vi "autofpga8.vi"() -> ()   [LabVIEW 2012]
uses:
  <vilib>/eio/EIONode/EIONode.xnode
  <vilib>/eio/EIOMethodNode/EIOMethodNode.xnode
  <vilib>/LabVIEW Targets/FPGA/RIO/nicrio_985x_controls.llb/CAN_IO_Frame Type.ctl
  <vilib>/LabVIEW Targets/FPGA/RIO/nicrio_985x_controls.llb/CAN_IO_Frame Cluster.ctl
  <vilib>/rvi/eio/common/nirviEmuTemplateMethod_errors.vi
  <vilib>/eio/EIOPropertyNode/EIOPropertyNode.xnode
  <vilib>/rvi/eio/common/nirviEmuTemplatePropertyGet_errors.vi
  <vilib>/rvi/eio/common/nirviEmuTemplatePropertyGet_noerrors.vi
  <vilib>/rvi/eio/common/nirviEmuTemplatePropertySet_errors.vi
  <vilib>/rvi/eio/common/nirviEmuTemplatePropertySet_noerrors.vi
  <vilib>/rvi/DataTransferAndStorage/Container/XNode/niFpgaContainer.xnode
  <vilib>/rvi/interface/RandomDataEmulation/nirviRandomDataFpgaReadWriteTemplate.vi
panel:
  out "Data":u8
  out "Is gps1 Connected":bool
  out "Connection error GPS 1":bool=TRUE
  out "GPS 1 clock":bool=TRUE
  out "DATA IMU 1":T1
  out "IMU Connection error":bool=TRUE
  out "Idle rpm":u8
  out "ODOMETERT_RL":u8
  out "WHEEL_FR":u8
  out "WHEEL_FRFL":u8
  out "WHEEL_FL":u8
  in  "16k":bool
  out "amp":fxp<+/-,16,5> format="%.13g"
  out "WHELL_RR":u8
  out "WHEEL_RRRL":u8
  out "WHEEL_RL":u8
  out "counter":bool=TRUE
  out "lock on":bool
  out "rpm":u16
  out "BREAK_ACT_TCU":u8
  out "VS_TCU 2":u8
  out "VS_TCU":u8
  out "VB":u8
  out "TPS":u8
  out "Vehicle speed":u8
  out "G_sel_disp":u8
  out "SAS_angle":i32
  out "SAS_angle_MDPS":i32
  out "OPT1_Read":bool
  in  "OPT1_Write":bool
  in  "OPT1_write enable":bool
  out "encoder":u16
  out "T Lim":bool
  in  "Buzz":bool
  out "CAN read":T2={"timestamp high"=0, "timestamp low"=0, "identifier"=0, "type"=enum."Data Frame", "info A"=0, "info B"=0, "data length"=0, "data"=[0, 0, 0, 0, 0, 0, 0, 0]} {"identifier" format="%x"; "timestamp high" format="%08x"; "timestamp low" format="%08x"; "data" format="%.0x"}
  in  "CAN Write":T2={"timestamp high"=0, "timestamp low"=0, "identifier"=1540, "type"=enum."Data Frame", "info A"=0, "info B"=0, "data length"=8, "data"=[0, 0, 0, 0, 0, 0, 0, 0]} {"identifier" format="%x"; "timestamp high" format="%08x"; "timestamp low" format="%08x"; "data" format="%.0x"}
  in  "read can":bool
  in  "B Pwm":u16
  in  "T Pwm":u16
  in  "Shift PWM":bool
  in  "B Dir":bool
  in  "B RDir":bool
  in  "Shift Dir":bool
  in  "T Dir":bool
  in  "T RDir":bool
  in  "Solenoid":bool
  out "Run":bool
  out "Auto":bool
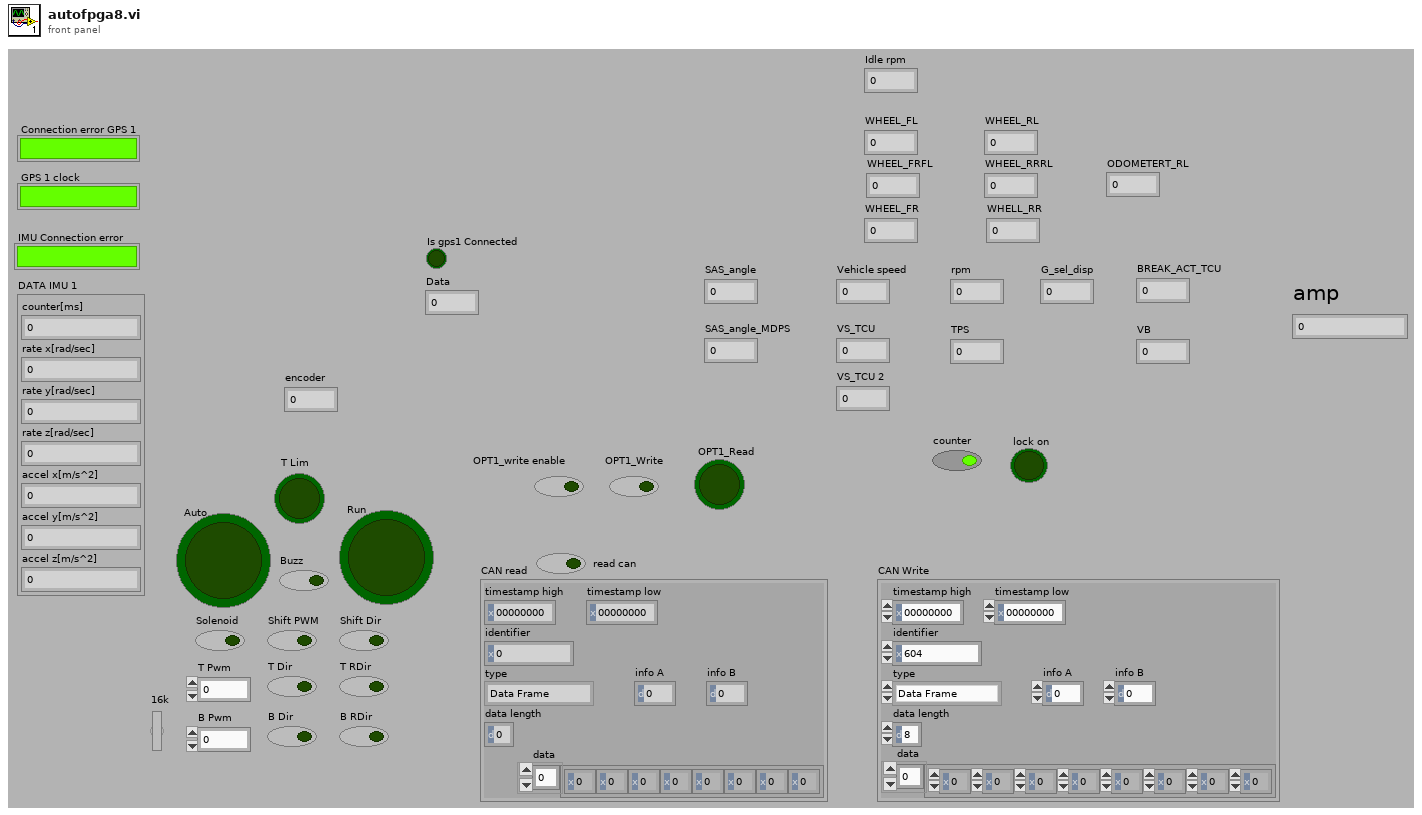
[diagram p1: front panel]
types:
  T1 = cluster{"counter[ms]":u16, "rate x[rad/sec]":i16, "rate y[rad/sec]":i16, "rate z[rad/sec]":i16, "accel x[m/s^2]":i16, "accel y[m/s^2]":i16, "accel z[m/s^2]":i16}
  T2 = typedef "CAN_IO_Frame Cluster.ctl" = cluster{"timestamp high":u32, "timestamp low":u32, "identifier":u32, "type":T3, "info A":u8, "info B":u8, "data length":u8, "data":u8[]}
  T3 = typedef "CAN_IO_Frame Type.ctl" = enum8{"Data Frame", "Remote Frame", "(reserved)", "(reserved) ", "(reserved)  ", "(reserved)   ", "Bus Error", "Transceiver Fault"}
  T4 = cluster{"data[0]":u8, "data[1]":u8, "data[2]":u8, "data[3]":u8, "data[4]":u8, "data[5]":u8, "data[6]":u8, "data[7]":u8}
  T5 = cluster{"[0]":void, "[1]":void, "[2]":void, "[3]":void, "[4]":void, "[5]":void, "[6]":void, "[7]":void, "[8]":void, "[9]":void, "[10]":void, "[11]":void, "[12]":void, "[13]":void}
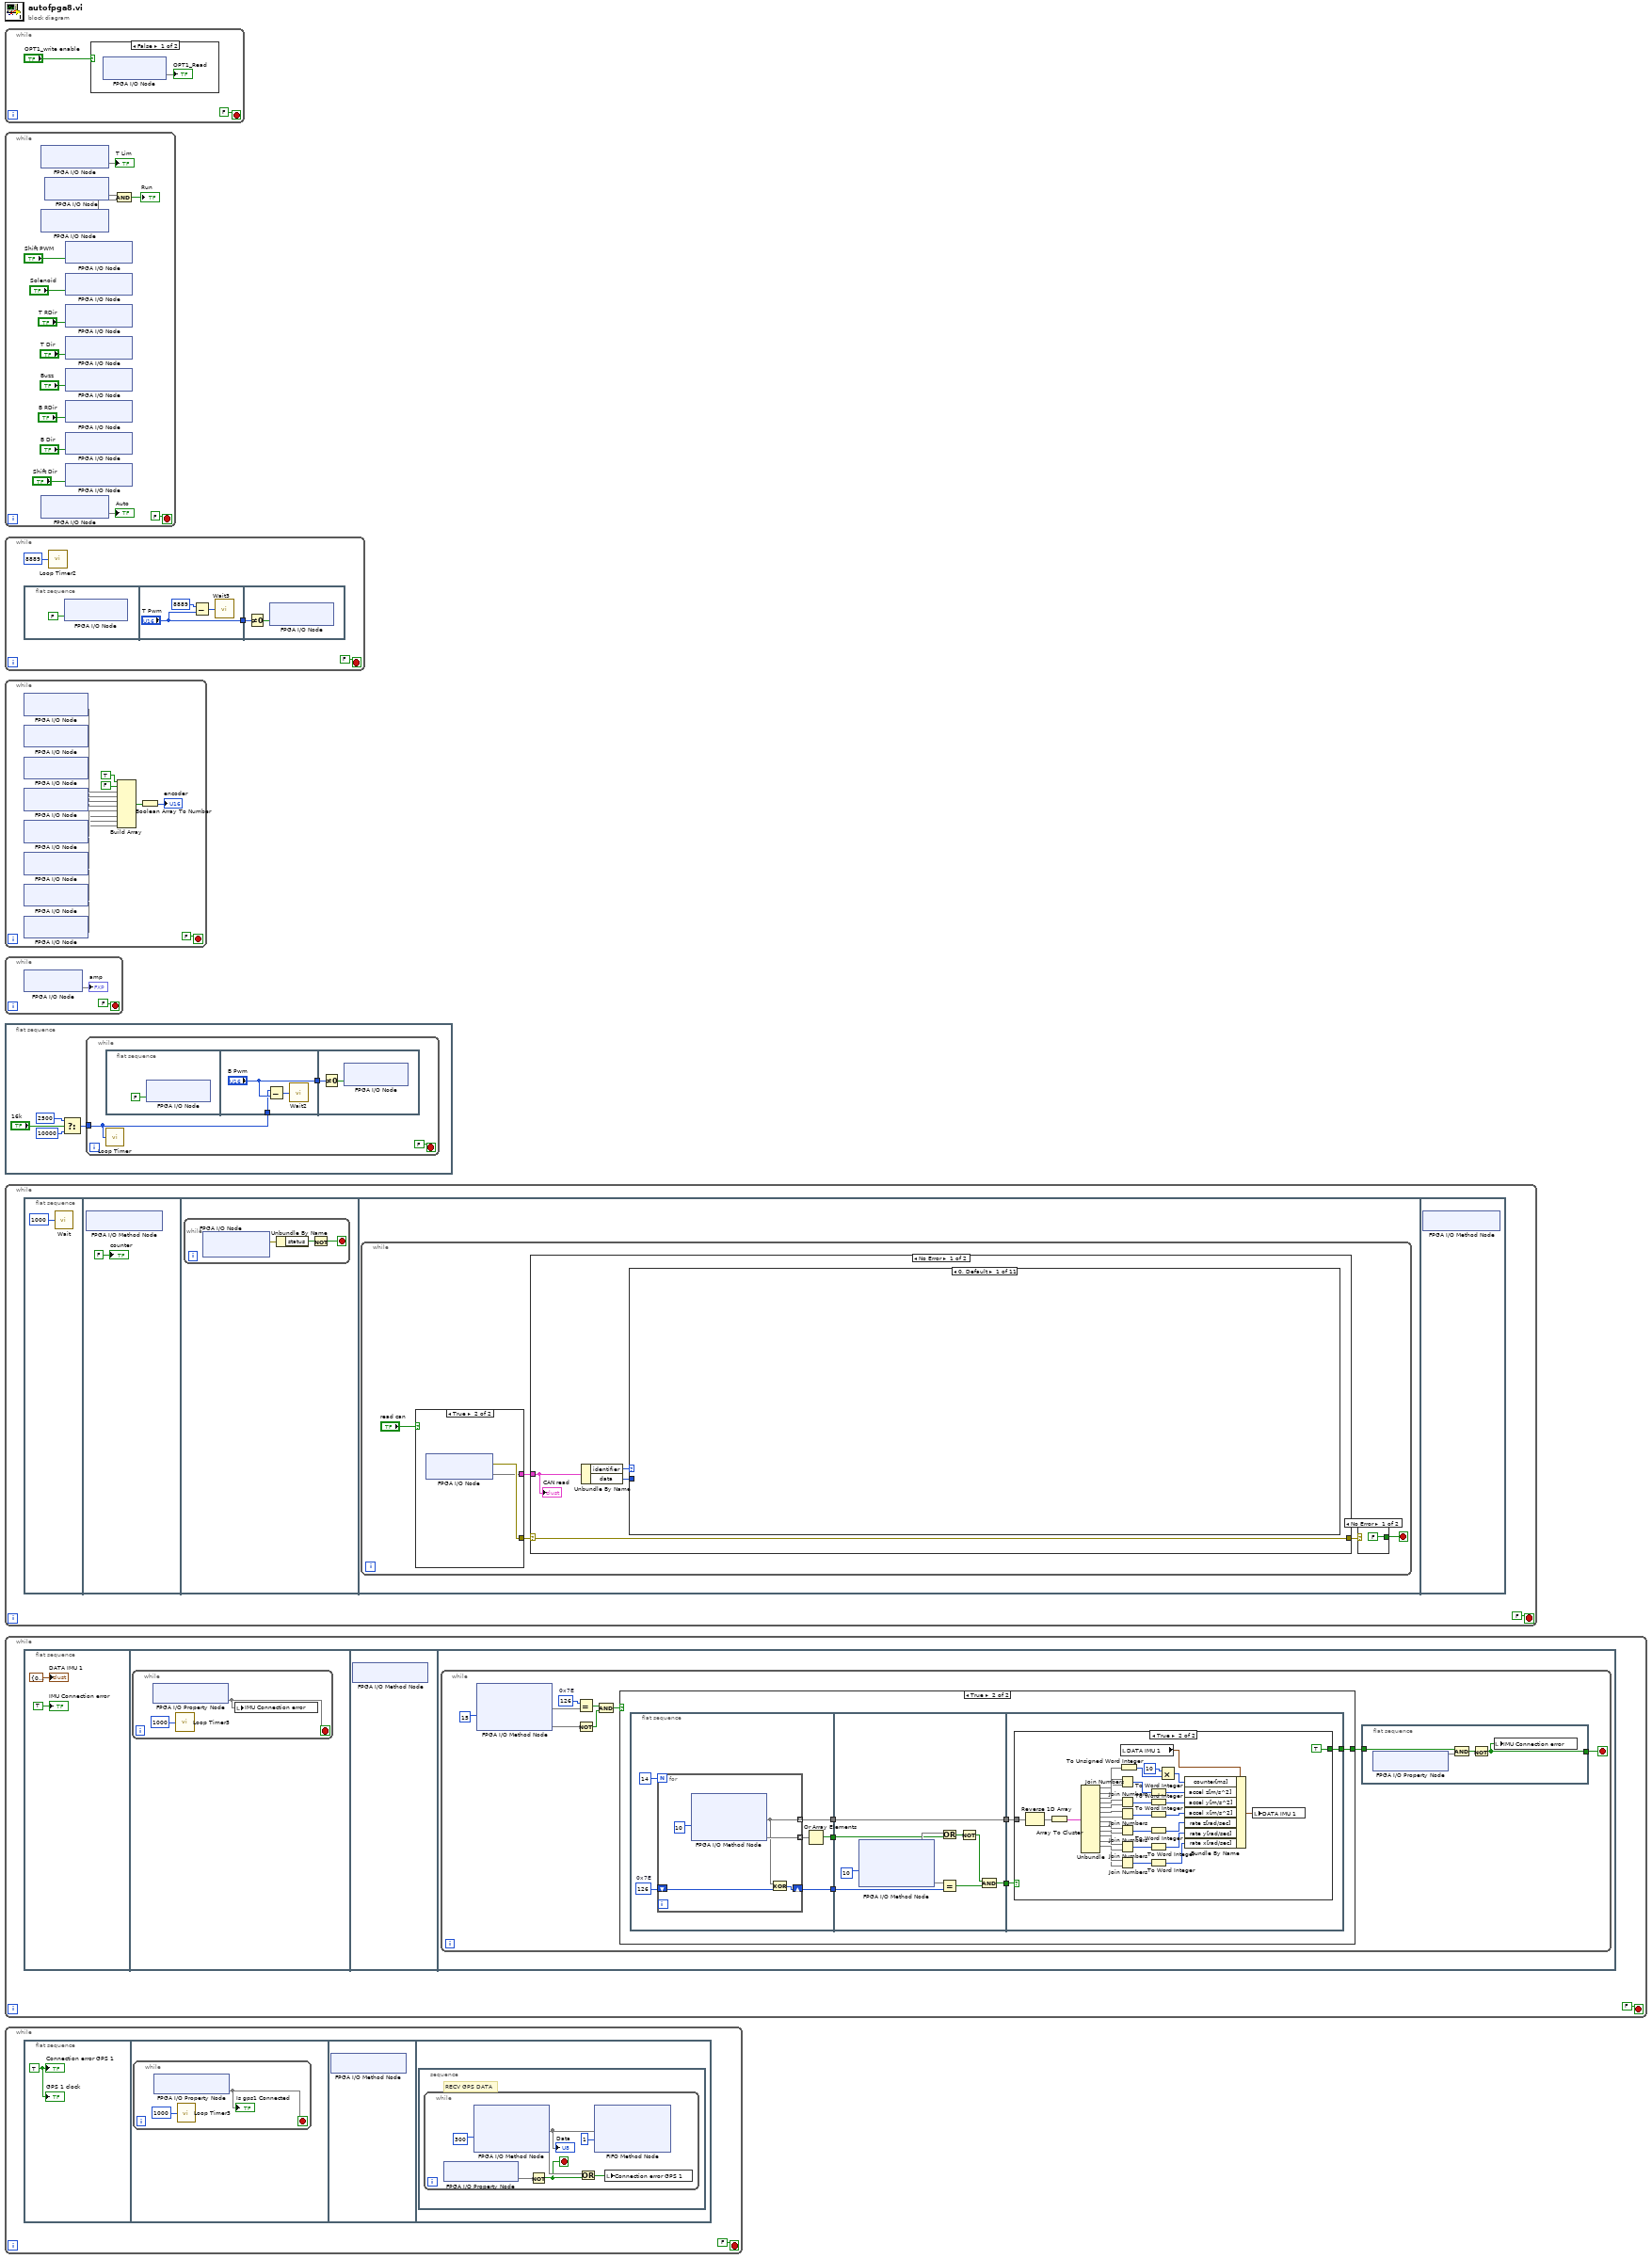
[diagram p0: block diagram]
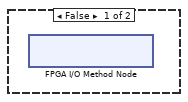
[diagram p3: hidden frame]
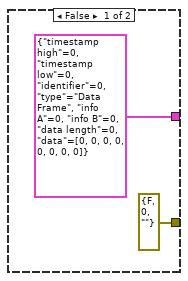
[diagram p4: hidden frame]
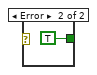
[diagram p5: hidden frame]
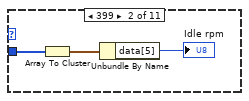
[diagram p6: hidden frame]
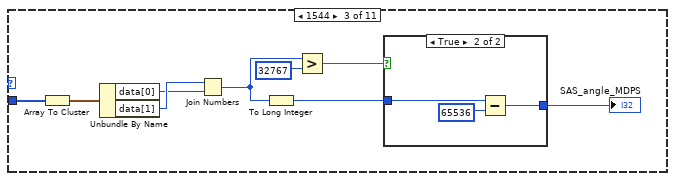
[diagram p7: hidden frame]
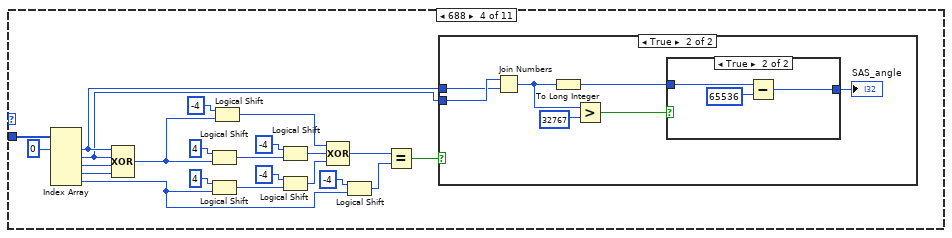
[diagram p9: hidden frame]
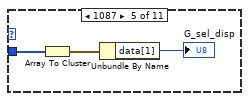
[diagram p12: hidden frame]
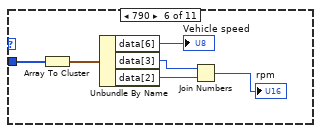
[diagram p13: hidden frame]
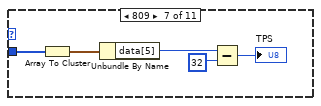
[diagram p14: hidden frame]
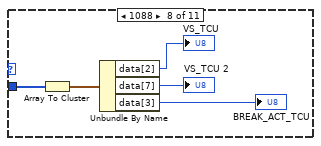
[diagram p15: hidden frame]
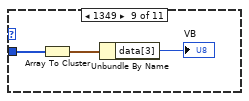
[diagram p16: hidden frame]
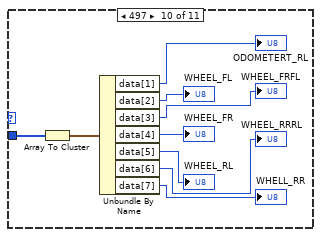
[diagram p17: hidden frame]
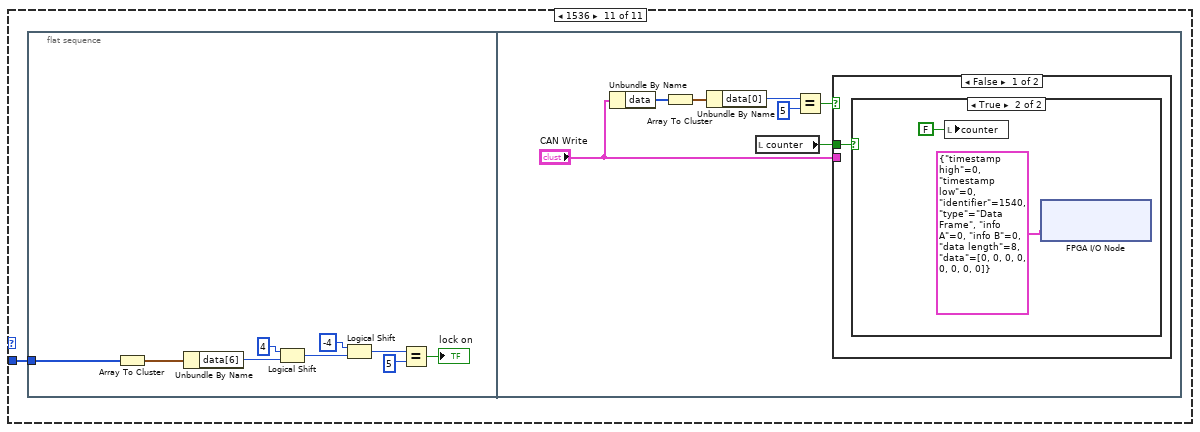
[diagram p18: hidden frame]
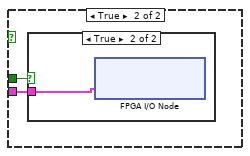
[diagram p20: hidden frame]
diagram:
  n1 = while {
    stop <- FALSE stop-if-true
    n2 = case shown="False" "OPT1_write enable" {
      frame False {
        n3 = xnode "FPGA I/O Node"() -> ("Mod1/DIO0"=→"OPT1_Read")  [unwired: 1 in, 1 out]
      }
      frame True {
        n4 = xnode "FPGA I/O Node"("Mod1/DIO0"="OPT1_Write") -> ()  [unwired: 1 in, 1 out]
      }
    }
  }
  n5 = while {
    stop <- FALSE stop-if-true
    n6 = xnode "FPGA I/O Node"() -> ("Mod1/DIO15"=→"T Lim")  [unwired: 1 in, 1 out]
    n7 = xnode "FPGA I/O Node"() -> ("Mod1/DIO12"=w7)  [unwired: 1 in, 1 out]
    n8 = xnode "FPGA I/O Node"() -> ("Mod1/DIO11"=→"Auto")  [unwired: 1 in, 1 out]
    n9 = xnode "FPGA I/O Node"() -> ("Mod1/DIO0"=w8)  [unwired: 1 in, 1 out]
    n10 = xnode "FPGA I/O Node"("Mod1/DIO19"="Shift PWM") -> ()  [unwired: 1 in, 1 out]
    n11 = xnode "FPGA I/O Node"("Mod1/DIO13"="Solenoid") -> ()  [unwired: 1 in, 1 out]
    n12 = xnode "FPGA I/O Node"("Mod1/DIO17"="T RDir") -> ()  [unwired: 1 in, 1 out]
    n13 = xnode "FPGA I/O Node"("Mod1/DIO18"="T Dir") -> ()  [unwired: 1 in, 1 out]
    n14 = xnode "FPGA I/O Node"("Mod1/DIO24"="Buzz") -> ()  [unwired: 1 in, 1 out]
    n15 = xnode "FPGA I/O Node"("Mod1/DIO22"="B RDir") -> ()  [unwired: 1 in, 1 out]
    n16 = xnode "FPGA I/O Node"("Mod1/DIO23"="B Dir") -> ()  [unwired: 1 in, 1 out]
    n17 = xnode "FPGA I/O Node"("Mod1/DIO20"="Shift Dir") -> ()  [unwired: 1 in, 1 out]
    n18 = And(x=w8, y=w7) -> (x .and. y?=→"Run":bool)
  }
  n19 = while {
    stop <- FALSE stop-if-true
    n20 = flat-sequence {
      tunnel: ["T Pwm"] -> w19
      tunnel: w19 -> [w27]
      frame #0 {
        n21 = xnode "FPGA I/O Node"("Mod4/DIO1"=FALSE ("Mod1/DIO16")) -> ()  [unwired: 1 in, 1 out]
      }
      frame #1 {
        n22 = Subtract(x=u16 8889, y="T Pwm") -> (x-y=w24:u16)
        n23 = call "Wait3"("Count(Ticks)"=w24) -> ()  [unwired: 1 out]
      }
      frame #2 {
        n24 = Not Equal To 0?(x=w27) -> (x != 0?=w26:bool)
        n25 = xnode "FPGA I/O Node"("Mod4/DIO1"=w26) -> ()  [unwired: 1 in, 1 out]
      }
    }
    n26 = call "Loop Timer2"("Count(Ticks)"=u16 8889) -> ()  [unwired: 1 out]
  }
  n27 = while {
    stop <- FALSE stop-if-true
    n28 = xnode "FPGA I/O Node"() -> ("Mod1/DIO2"=w40)  [unwired: 1 in, 1 out]
    n29 = xnode "FPGA I/O Node"() -> ("Mod1/DIO3"=w39)  [unwired: 1 in, 1 out]
    n30 = xnode "FPGA I/O Node"() -> ("Mod1/DIO4"=w38)  [unwired: 1 in, 1 out]
    n31 = xnode "FPGA I/O Node"() -> ("Mod1/DIO5"=w37)  [unwired: 1 in, 1 out]
    n32 = xnode "FPGA I/O Node"() -> ("Mod1/DIO6"=w36)  [unwired: 1 in, 1 out]
    n33 = xnode "FPGA I/O Node"() -> ("Mod1/DIO7"=w35)  [unwired: 1 in, 1 out]
    n34 = xnode "FPGA I/O Node"() -> ("Mod1/DIO8"=w34)  [unwired: 1 in, 1 out]
    n35 = xnode "FPGA I/O Node"() -> ("Mod1/DIO9"=w33)  [unwired: 1 in, 1 out]
    n36 = Build Array(TRUE ("element"), FALSE ("element"), w40, w39, w38, w37, w36, w35, w34, w33) -> (w31:bool[])
    n37 = Boolean Array To Number(Boolean array=w31) -> (number=→"encoder":u32)
  }
  n38 = while {
    stop <- FALSE stop-if-true
    n39 = xnode "FPGA I/O Node"() -> ("Mod3/AI7"=→"amp")  [unwired: 1 in, 1 out]
  }
  n40 = flat-sequence {
    frame #0 {
      n41 = Select(t=u16 2500, s="16k", f=u16 10000) -> (s? t:f=w43:u16)
      n42 = while {
        tunnel: w43 -> [w47]
        stop <- FALSE stop-if-true
        n43 = flat-sequence {
          tunnel: ["B Pwm"] -> w49
          tunnel: w47 -> [w51]
          tunnel: w49 -> [w55]
          frame #0 {
            n44 = xnode "FPGA I/O Node"("Mod4/DIO0"=FALSE ("Mod1/DIO21")) -> ()  [unwired: 1 in, 1 out]
          }
          frame #1 {
            n45 = Subtract(x=w51, y="B Pwm") -> (x-y=w53:u16)
            n46 = call "Wait2"("Count(Ticks)"=w53) -> ()  [unwired: 1 out]
          }
          frame #2 {
            n47 = Not Equal To 0?(x=w55) -> (x != 0?=w54:bool)
            n48 = xnode "FPGA I/O Node"("Mod4/DIO0"=w54) -> ()  [unwired: 1 in, 1 out]
          }
        }
        n49 = call "Loop Timer"("Count(Ticks)"=w47) -> ()  [unwired: 1 out]
      }
    }
  }
  n50 = while {
    stop <- FALSE stop-if-true
    n51 = flat-sequence {
      frame #0 {
        n52 = call "Wait"("Count(mSec)"=u16 1000) -> ()  [unwired: 1 out]
      }
      frame #1 {
        n53 = xnode "FPGA I/O Method Node"() -> ()  [unwired: 2 in, 2 out]
        "counter" <- FALSE
      }
      frame #2 {
        n54 = while {
          stop <- w59 stop-if-true
          n55 = xnode "FPGA I/O Node"() -> ("error out"=w61:errorcluster)  [unwired: 2 in, 2 out]
          n56 = Unbundle By Name(w61) -> ("status"=w60:bool)
          n57 = Not(x=w60) -> (.not. x?=w59:bool)
        }
      }
      frame #3 {
        n58 = while {
          stop <- w62 stop-if-true
          n59 = case shown="True" "read can" {
            tunnel: [errorcluster {"status"=FALSE, "code"=0, "source"=""} ("error out") w70] -> w66
            tunnel: [T2 {"timestamp high"=0, "timestamp low"=0, "identifier"=0, "type"=enum."Data Frame", "info A"=0, "info B"=0, "data length"=0, "data"=[0, 0, 0, 0, 0, 0, 0, 0]} ("Mod3/CAN0") w69] -> w65
            frame False {
            }
            frame True {
              n60 = xnode "FPGA I/O Node"() -> ("error out"=w70:errorcluster, "Mod2/CAN0"=w69)  [unwired: 2 in, 1 out]
            }
          }
          n61 = case shown="No Error" w66 {
            selector: w66 -> [w73 w181]
            tunnel: w65 -> [w76 _]
            tunnel: [w73 w181] -> w64
            frame No Error {
              n62 = Unbundle By Name(w76) -> ("identifier"=w75:u32, "data"=w74:u8[])
              n63 = case shown="0, Default" w75 {
                tunnel: w74 -> [_ w78 w87 w93 w128 w133 w138 w143 w146 w155 w157]
                frame 0, Default {
                }
                frame 399 {
                  n64 = Array To Cluster(array=w78) -> (cluster=w79:T4)
                  n65 = Unbundle By Name(w79) -> ("data[5]"=→"Idle rpm":u8)
                }
                frame 1544 {
                  n66 = Array To Cluster(array=w87) -> (cluster=w88:T4)
                  n67 = Unbundle By Name(w88) -> ("data[0]"=w85:u8, "data[1]"=w86:u8)
                  n68 = Join Numbers(hi=w86, lo=w85) -> ((hi.lo)=w82:u16)
                  n69 = To Long Integer(number=w82) -> (32bit integer=w81:i32)
                  n70 = Greater?(x=w82, y=u16 32767) -> (0:w83:bool)
                  n71 = case shown="True" w83 {
                    tunnel: w81 -> [w89 w90]
                    tunnel: [w89 w91] -> w80
                    frame False {
                    }
                    frame True {
                      n72 = Subtract(x=w90, y=65536) -> (x-y=w91:i32)
                    }
                  }
                  "SAS_angle_MDPS" <- w80
                }
                frame 688 {
                  n73 = Index Array(array=w93, index #1=0 ("index")) -> (element #1=w98:u8, element #2=w97:u8, element #3=w96:u8, element #4=w95:u8, element #5=w94:u8)  [unwired: 4 in]
                  n74 = Compound Arithmetic op=XOR(w98, w97, w96, w95) -> (w114:u8)
                  n75 = Logical Shift(y=i8 4, x=w114) -> (x << y=w113:u8)
                  n76 = Logical Shift(y=i8 4, x=w94) -> (x << y=w106:u8)
                  n77 = Logical Shift(y=i8 -4, x=w114) -> (x << y=w107:u8)
                  n78 = Logical Shift(y=i8 -4, x=w113) -> (x << y=w108:u8)
                  n79 = Logical Shift(y=i8 -4, x=w106) -> (x << y=w101:u8)
                  n80 = Compound Arithmetic op=XOR(w107, w108, w101) -> (w109:u8)
                  n81 = Logical Shift(y=i8 -4, x=w94) -> (x << y=w102:u8)
                  n82 = Equal?(x=w109, y=w102) -> (x = y?=w100:bool)
                  n83 = case shown="True" w100 {
                    tunnel: w97 -> [_ w121]
                    tunnel: w98 -> [_ w120]
                    frame False {
                    }
                    frame True {
                      n84 = Join Numbers(hi=w121, lo=w120) -> ((hi.lo)=w117:u16)
                      n85 = To Long Integer(number=w117) -> (32bit integer=w116:i32)
                      n86 = Greater?(x=w117, y=u16 32767) -> (0:w118:bool)
                      n87 = case shown="True" w118 {
                        tunnel: w116 -> [w122 w124]
                        tunnel: [w122 w123] -> w115
                        frame False {
                        }
                        frame True {
                          n88 = Subtract(x=w124, y=65536) -> (x-y=w123:i32)
                        }
                      }
                      "SAS_angle" <- w115
                    }
                  }
                }
                frame 1087 {
                  n89 = Array To Cluster(array=w128) -> (cluster=w127:T4)
                  n90 = Unbundle By Name(w127) -> ("data[1]"=→"G_sel_disp":u8)
                }
                frame 790 {
                  n91 = Array To Cluster(array=w133) -> (cluster=w134:T4)
                  n92 = Unbundle By Name(w134) -> ("data[6]"=→"Vehicle speed":u8, "data[3]"=w131:u8, "data[2]"=w130:u8)
                  n93 = Join Numbers(hi=w131, lo=w130) -> ((hi.lo)=→"rpm":u16)
                }
                frame 809 {
                  n94 = Array To Cluster(array=w138) -> (cluster=w139:T4)
                  n95 = Unbundle By Name(w139) -> ("data[5]"=w137:u8)
                  n96 = Subtract(x=w137, y=u8 32) -> (x-y=→"TPS":u8)
                }
                frame 1088 {
                  n97 = Array To Cluster(array=w143) -> (cluster=w144:T4)
                  n98 = Unbundle By Name(w144) -> ("data[2]"=→"VS_TCU":u8, "data[7]"=→"VS_TCU 2":u8, "data[3]"=→"BREAK_ACT_TCU":u8)
                }
                frame 1349 {
                  n99 = Array To Cluster(array=w146) -> (cluster=w147:T4)
                  n100 = Unbundle By Name(w147) -> ("data[3]"=→"VB":u8)
                }
                frame 497 {
                  n101 = Array To Cluster(array=w155) -> (cluster=w156:T4)
                  n102 = Unbundle By Name(w156) -> ("data[1]"=→"ODOMETERT_RL":u8, "data[2]"=→"WHEEL_FL":u8, "data[3]"=→"WHEEL_FRFL":u8, "data[4]"=→"WHEEL_FR":u8, "data[5]"=→"WHEEL_RL":u8, "data[6]"=→"WHEEL_RRRL":u8, "data[7]"=→"WHELL_RR":u8)
                }
                frame 1536 {
                  n103 = flat-sequence {
                    tunnel: w157 -> [w166]
                    frame #0 {
                      n104 = Array To Cluster(array=w166) -> (cluster=w165:T4)
                      n105 = Unbundle By Name(w165) -> ("data[6]"=w164:u8)
                      n106 = Logical Shift(y=i8 4, x=w164) -> (x << y=w163:u8)
                      n107 = Logical Shift(y=i8 -4, x=w163) -> (x << y=w160:u8)
                      n108 = Equal?(x=w160, y=u8 5) -> (x = y?=→"lock on":bool)
                    }
                    frame #1 {
                      n109 = Unbundle By Name("CAN Write") -> ("data"=w171:u8[])
                      n110 = Array To Cluster(array=w171) -> (cluster=w170:T4)
                      n111 = Unbundle By Name(w170) -> ("data[0]"=w169:u8)
                      n112 = local read "counter"() -> (w167:bool)
                      n113 = Equal?(x=w169, y=u8 5) -> (x = y?=w173:bool)
                      n114 = case shown="False" w173 {
                        tunnel: "CAN Write" -> [_ w178]
                        tunnel: w167 -> [w174 w177]
                        frame False {
                          n115 = case shown="True" w174 {
                            frame False {
                            }
                            frame True {
                              n116 = local write "counter"(FALSE ("counter")) -> ()
                              n117 = xnode "FPGA I/O Node"("Mod2/CAN0"=T2 {"timestamp high"=0, "timestamp low"=0, "identifier"=1540, "type"=enum."Data Frame", "info A"=0, "info B"=0, "data length"=8, "data"=[0, 0, 0, 0, 0, 0, 0, 0]} ("CAN Write")) -> ()  [unwired: 2 in, 2 out]
                            }
                          }
                        }
                        frame True {
                          n118 = case shown="True" w177 {
                            tunnel: w178 -> [_ w180]
                            frame False {
                              n119 = local write "counter"(TRUE ("counter")) -> ()
                            }
                            frame True {
                              n120 = xnode "FPGA I/O Node"("Mod2/CAN0"=w180) -> ()  [unwired: 2 in, 2 out]
                            }
                          }
                        }
                      }
                    }
                  }
                }
              }
              "CAN read" <- w76
            }
            frame Error {
            }
          }
          n121 = case shown="No Error" w64 {
            tunnel: [FALSE ("can_ini") TRUE ("can_ini")] -> w62
            frame No Error {
            }
            frame Error {
            }
          }
        }
      }
      frame #4 {
        n122 = xnode "FPGA I/O Method Node"() -> ()  [unwired: 2 in, 2 out]
      }
    }
  }
  n123 = while {
    stop <- FALSE stop-if-true
    n124 = flat-sequence {
      frame #0 {
        "DATA IMU 1" <- T1 {"counter[ms]"=0, "rate x[rad/sec]"=0, "rate y[rad/sec]"=0, "rate z[rad/sec]"=0, "accel x[m/s^2]"=0, "accel y[m/s^2]"=0, "accel z[m/s^2]"=0} ("DATA IMU 1")
        "IMU Connection error" <- TRUE ("IMU Connection error")
      }
      frame #1 {
        n125 = while {
          stop <- w185 stop-if-true
          n126 = xnode "FPGA I/O Property Node"() -> ("Is Connected"=w185)  [unwired: 1 in, 1 out]
          n127 = call "Loop Timer5"("Count(mSec)"=u32 1000) -> ()  [unwired: 1 out]
          n128 = local write "IMU Connection error"(w185) -> ()
        }
      }
      frame #2 {
        n129 = xnode "FPGA I/O Method Node"() -> ()  [unwired: 1 in, 1 out]
      }
      frame #3 {
        n130 = while {
          stop <- w187 stop-if-true
          w189 = u8 126  # 0x7E
          n131 = xnode "FPGA I/O Method Node"("Timeout (ms)"=15) -> ("Data"=w190, "Timed Out"=w194)  [unwired: 1 in, 1 out]
          n132 = Equal?(x=w189, y=w190) -> (x = y?=w193:bool)
          n133 = Not(x=w194) -> (.not. x?=w192:bool)
          n134 = And(x=w193, y=w192) -> (x .and. y?=w191:bool)
          n135 = case shown="True" w191 {
            tunnel: [_ w201] -> w188
            frame False {
            }
            frame True {
              n136 = flat-sequence {
                tunnel: [w209] -> w205
                tunnel: [w208] -> w203
                tunnel: [w206] -> w200
                tunnel: w205 -> [w226]
                tunnel: [w226] -> w204
                tunnel: w203 -> [w219]
                tunnel: [w221] -> w202
                tunnel: w200 -> [w223]
                tunnel: w204 -> [w229]
                tunnel: w202 -> [w228]
                tunnel: [w227] -> w201
                frame #0 {
                  w210 = u8 126  # 0x7E
                  n137 = for {
                    N: 14 -> [_]
                    tunnel: [w213] -> w209 mode=indexing
                    shift-right: [w215] -> w208
                    shift-left: w210 -> [w212]
                    tunnel: [w214] -> w207 mode=indexing
                    n138 = xnode "FPGA I/O Method Node"("Timeout (ms)"=10) -> ("Data"=w213, "Timed Out"=w214)  [unwired: 1 in, 1 out]
                    n139 = Exclusive Or(1:w212, 2:w213) -> (0:w215:u8)
                  }
                  n140 = Or Array Elements(Boolean array=w207) -> (logical OR=w206:bool)
                }
                frame #1 {
                  n141 = xnode "FPGA I/O Method Node"("Timeout (ms)"=10) -> ("Data"=w220, "Timed Out"=w224)  [unwired: 1 in, 1 out]
                  n142 = Or(x=w224, y=w223) -> (x .or. y?=w222:bool)
                  n143 = Equal?(x=w220, y=w219) -> (x = y?=w218:bool)
                  n144 = Not(x=w222) -> (.not. x?=w217:bool)
                  n145 = And(x=w217, y=w218) -> (x .and. y?=w221:bool)
                }
                frame #2 {
                  n146 = case shown="True" w228 {
                    tunnel: w229 -> [_ w263]
                    tunnel: [_ TRUE ("IMU Connection error")] -> w227
                    frame False {
                      n147 = xnode "FPGA I/O Method Node"() -> ()  [unwired: 1 in, 1 out]
                    }
                    frame True {
                      n148 = Reverse 1D Array(array=w263) -> (reversed array=w262:void[])
                      n149 = Array To Cluster(array=w262) -> (cluster=w261:T5)
                      n150 = Unbundle(w261) -> ("[0]"=w240, "[1]"=w260, "[2]"=w259, "[3]"=w258, "[4]"=w257, "[5]"=w256, "[6]"=w255, "[7]"=w254, "[8]"=w253, "[9]"=w252, "[10]"=w251, "[11]"=w250, "[12]"=w249)  [unwired: 1 out]
                      n151 = Join Numbers(hi=w260, lo=w259) -> ((hi.lo)=w248:u32)
                      n152 = Join Numbers(hi=w258, lo=w257) -> ((hi.lo)=w247:u32)
                      n153 = Join Numbers(hi=w256, lo=w255) -> ((hi.lo)=w246:u32)
                      n154 = Join Numbers(hi=w254, lo=w253) -> ((hi.lo)=w245:u32)
                      n155 = Join Numbers(hi=w252, lo=w251) -> ((hi.lo)=w244:u32)
                      n156 = Join Numbers(hi=w250, lo=w249) -> ((hi.lo)=w243:u32)
                      n157 = To Unsigned Word Integer(number=w240) -> (unsigned 16bit integer=w239:u16)
                      n158 = local read "DATA IMU 1"() -> (w241:T1)
                      n159 = To Word Integer(number=w248) -> (16bit integer=w236:i16)
                      n160 = To Word Integer(number=w247) -> (16bit integer=w235:i16)
                      n161 = To Word Integer(number=w246) -> (16bit integer=w234:i16)
                      n162 = To Word Integer(number=w245) -> (16bit integer=w233:i16)
                      n163 = To Word Integer(number=w244) -> (16bit integer=w232:i16)
                      n164 = To Word Integer(number=w243) -> (16bit integer=w231:i16)
                      n165 = Multiply(x=u16 10, y=w239) -> (x*y=w237:u16)
                      n166 = Bundle By Name(cluster=w241, "counter[ms]"=w237, "accel z[m/s^2]"=w236, "accel y[m/s^2]"=w235, "accel x[m/s^2]"=w234, "rate z[rad/sec]"=w233, "rate y[rad/sec]"=w232, "rate x[rad/sec]"=w231) -> (w242:T1)
                      n167 = local write "DATA IMU 1"(w242) -> ()
                    }
                  }
                }
              }
            }
          }
          n168 = flat-sequence {
            tunnel: w188 -> [w198]
            tunnel: [w196] -> w187
            frame #0 {
              n169 = xnode "FPGA I/O Property Node"() -> ("Is Connected"=w199)  [unwired: 1 in, 1 out]
              n170 = And(x=w198, y=w199) -> (x .and. y?=w197:bool)
              n171 = Not(x=w197) -> (.not. x?=w196:bool)
              n172 = local write "IMU Connection error"(w196) -> ()
            }
          }
        }
      }
    }
  }
  n173 = while {
    stop <- FALSE stop-if-true
    n174 = flat-sequence {
      frame #0 {
        w265 = TRUE ("GPS 1 Connection error")
        "Connection error GPS 1" <- w265
        "GPS 1 clock" <- w265
      }
      frame #1 {
        n175 = while {
          stop <- w267 stop-if-true
          n176 = xnode "FPGA I/O Property Node"() -> ("Is Connected"=w267)  [unwired: 1 in, 1 out]
          "Is gps1 Connected" <- w267
          n177 = call "Loop Timer3"("Count(mSec)"=u32 1000) -> ()  [unwired: 1 out]
        }
      }
      frame #2 {
        n178 = xnode "FPGA I/O Method Node"() -> ()  [unwired: 1 in, 1 out]
      }
      frame #3 {
        n179 = stacked-sequence {
          frame #0 {
            # "RECV GPS DATA"
            n180 = while {
              stop <- w268 stop-if-true
              n181 = xnode "FPGA I/O Property Node"() -> ("Is Connected"=w274)  [unwired: 1 in, 1 out]
              n182 = xnode "FPGA I/O Method Node"("Timeout (ms)"=300) -> ("Data"=w270, "Timed Out"=w269)  [unwired: 1 in, 1 out]
              "Data" <- w270
              n183 = Not(x=w274) -> (.not. x?=w268:bool)
              n184 = Or(x=w269, y=w268) -> (x .or. y?=w271:bool)
              n185 = xnode ("FIFO Method Node")("Element"=w270, "Timeout"=1) -> ()  [unwired: 1 in, 2 out]
              n186 = local write "Connection error GPS 1"(w271) -> ()
            }
          }
        }
      }
    }
  }
